vi "WriteConfigure.vi"(8 "error in (no error)":errorcluster, 10 "Para":string[][](array[string]), 11 "section":string caption="段") -> (0 "error out":errorcluster)   [LabVIEW 2016, in "DGUS.lvlib"]
uses:
  DGUS.lvlib
  <vilib>/Utility/config.llb/Write Key (String).vi
  <vilib>/Utility/config.llb/NI_LVConfig.lvlib
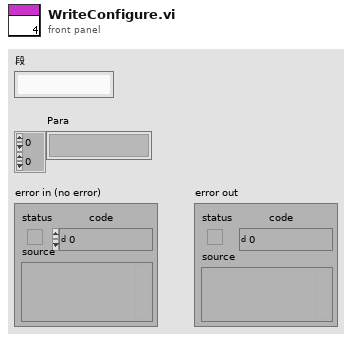
[diagram p1: front panel]
types:
  T1 = typedef "NI_LVConfig.lvlib/Config Data RefNum.ctl" = refnum<k1>
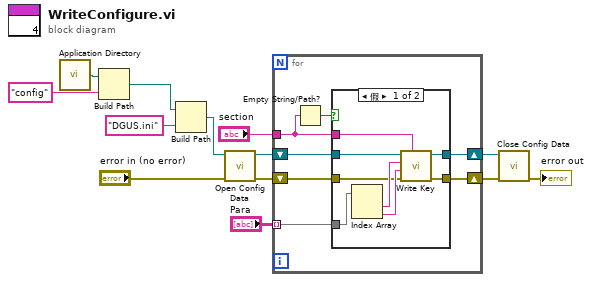
[diagram p0: block diagram]
diagram:
  n1 = call <vilib>:"Application Directory.vi"() -> ("Application Directory"=w7:path)
  n2 = Build Path(base path=w7, name or relative path="config" ("名称或相对路径")) -> (appended path=w5:path)
  n3 = Build Path(base path=w5, name or relative path="DGUS.ini" ("名称或相对路径")) -> (appended path=w3:path)
  n4 = call <vilib>:"Open Config Data.vi"("error in (no error)"="error in (no error)", "configuration file path"=w3) -> ("error out"=w11:errorcluster, "refnum"=w13:T1)  [unwired: 7 in, 1 out]
  n5 = for {
    tunnel: "Para" -> [w19] mode=indexing
    shift-right: [w16] -> w10
    shift-left: w13 -> [w20]
    shift-right: [w17] -> w9
    shift-left: w11 -> [w18]
    tunnel: "section" -> [w15]
    n6 = Empty String/Path?(string/path=w15) -> (empty?=w14:bool)
    n7 = case shown="假" w14 {
      tunnel: w20 -> [w28 w30]
      tunnel: w19 -> [w27 _]
      tunnel: w18 -> [w24 w29]
      tunnel: [w23 w29] -> w17
      tunnel: [w22 w30] -> w16
      tunnel: w15 -> [w21 _]
      frame False {
        n8 = Index Array(array=w27) -> (element #1=w26:string, element #2=w25:string)  [unwired: 2 in]
        n9 = call-poly <vilib>:"Write Key.vi"("section"=w21, "error in (no error)"=w24, "value"=w25, "key"=w26, "refnum"=w28) -> ("error out"=w23:errorcluster, "refnum out"=w22:T1)  [unwired: 4 in, 1 out]
      }
      frame True {
      }
    }
  }
  n10 = call <vilib>:"Close Config Data.vi"("error in (no error)"=w9, "refnum"=w10) -> ("error out"=→"error out":errorcluster)  [unwired: 8 in, 1 out]
